vi "ChannelASF.vi"(11 "ASF":dbl format="%.3f") -> (3 "ASF in hex":u32 format="%x")   [LabVIEW 2016]
panel:
  # "ASF"
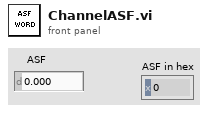
[diagram p1: front panel]
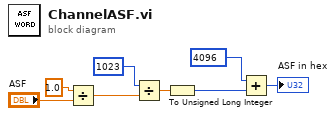
[diagram p0: block diagram]
diagram:
  n1 = Divide(x=1.0, y="ASF") -> (x/y=w1:dbl)
  n2 = Divide(x=u32 1023, y=w1) -> (x/y=w4:dbl)
  n3 = To Unsigned Long Integer(number=w4) -> (unsigned 32bit integer=w7:u32)
  n4 = Add(x=u32 4096, y=w7) -> (x+y=→"ASF in hex":u32)
